vi "PH_Beckhoff_PPMA-Rods.handle Digital Inputs.vi"(0 "i ref in":refnum<vi>, 2 "States":T2(array[cluster]) {"Status" items=["no info", "off/false/out", "on/true/in", "Failure", "Alarm", "Status 1", "Status 2", "Status 3"]}, 3 "Digital Inputs":T3, 5 "error in":errorcluster) -> (14 "i ref out":refnum<vi>, 19 "error out":errorcluster)   [LabVIEW 2014, in "PH_Beckhoff_PPMA-Rods.lvlib"]
doc: "This VI sets the digital Input GUI elements which is whether the rods ar up or not."
uses:
  PH_Beckhoff_PPMA-Rods.lvlib
  PH_Beckhoff/PH_Beckhoff.Digital Inputs.ctl
  PH_Basics/PH_StatusHandler/PH_StatusHandler.Status.ctl
  PH_Basics/PH_StatusHandler/PH_StatusHandler.lvlib
  PH_Beckhoff/PH_Beckhoff.lvlib
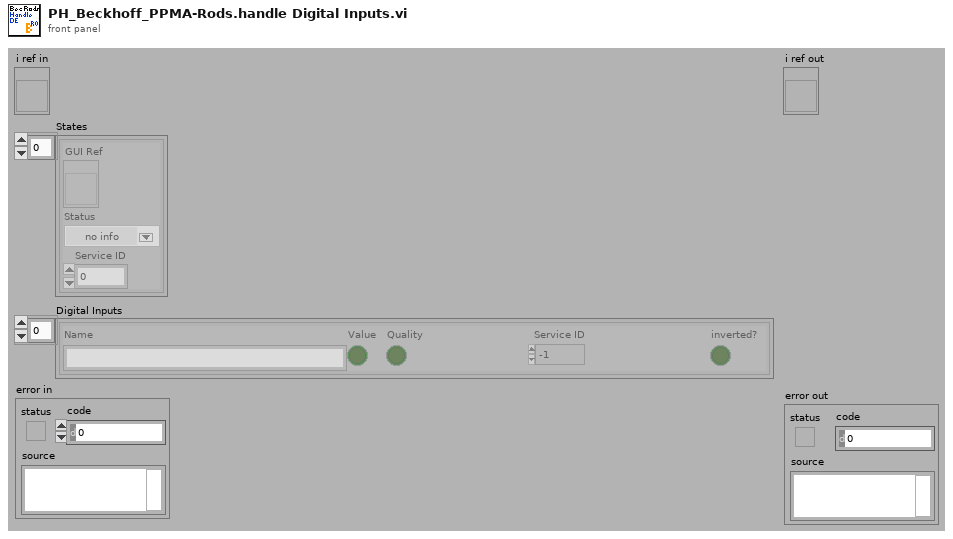
[diagram p1: front panel]
types:
  T1 = typedef "PH_StatusHandler.lvlib/PH_StatusHandler.Status.ctl" = i16
  T2 = cluster{"GUI Ref":refnum<vi>, "Status":T1, "Service ID":i32}[]
  T3 = typedef "PH_Beckhoff.lvlib/PH_Beckhoff.Digital Inputs.ctl" = cluster{"Name":string, "Value":bool, "Quality":bool, "Service ID":i32, "inverted?":bool}[]
  T4 = typedef "PH_Beckhoff_PPMA-Rods.lvlib/PH_Beckhoff_PPMA-Rods.i attribute.ctl" = cluster{"Input Up GUI Refs":refnum<vi>[], "Output GUI Refs":cluster{"Rod A up":refnum<vi>, "Rod B up":refnum<vi>, "Warnlamp orange":refnum<vi>, "Warnlamp green":refnum<vi>}, "States":cluster{"GUI Ref":refnum<vi>, "Status":T1, "Service ID":i32}[], "Input GUI Refs":cluster{"earth ok":refnum<vi>, "door locked K1":refnum<vi>, "door locked K2":refnum<vi>, "valve closed":refnum<vi>}}
  T5 = cluster{"GUI Ref":refnum<vi>, "Status":T1, "Service ID":i32}
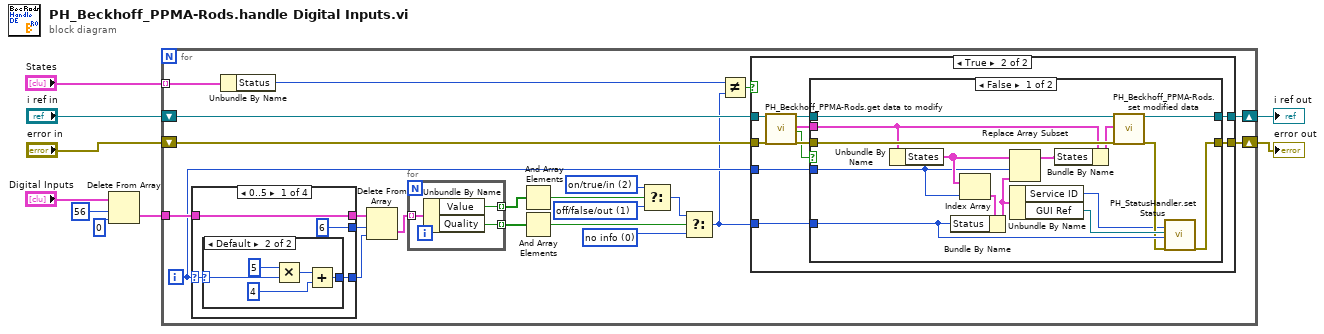
[diagram p0: block diagram]
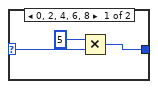
[diagram p4: hidden frame]
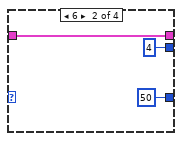
[diagram p5: hidden frame]
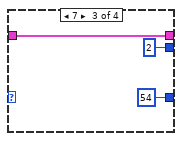
[diagram p6: hidden frame]
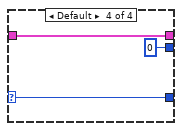
[diagram p7: hidden frame]
diagram:
  n1 = Delete From Array(array="Digital Inputs", length=56, index=0) -> (deleted portion=w1:T3)  [unwired: 1 out]
  n2 = for {
    shift-right: [w17] -> w7
    shift-left: "error in" -> [w31]
    tunnel: "States" -> [w30] mode=indexing
    tunnel: w1 -> [w29]
    shift-right: [w16] -> w3
    shift-left: "i ref in" -> [w15]
    i -> [w14]
    w19 = T1 1 items=["no info", "off/false/out", "on/true/in", "Failure", "Alarm", "Status 1", "Status 2", "Status 3"] ("f")
    w20 = T1 2 items=["no info", "off/false/out", "on/true/in", "Failure", "Alarm", "Status 1", "Status 2", "Status 3"] ("Status")
    w24 = T1 0 items=["no info", "off/false/out", "on/true/in", "Failure", "Alarm", "Status 1", "Status 2", "Status 3"] ("Status")
    n3 = case shown="0..5" w14 {
      selector: w14 -> [w64 _ _ w82]
      tunnel: w29 -> [w67 w78 w81 w84]
      tunnel: [w67 w78 w81 w84] -> w28
      tunnel: [6 ("length") 4 ("length") 2 ("length") 0 ("length")] -> w27
      tunnel: [w65 50 54 w82] -> w13
      frame 0..5 {
        n4 = case shown="Default" w64 {
          selector: w64 -> [w68 w74]
          tunnel: [w69 w73] -> w65
          frame 0, 2, 4, 6, 8 {
            n5 = Multiply(x=5 ("index"), y=w68) -> (x*y=w69:i32)
          }
          frame Default {
            n6 = Multiply(x=5 ("index"), y=w74) -> (x*y=w72:i32)
            n7 = Add(x=w72, y=4) -> (x+y=w73:i32)
          }
        }
      }
      frame 6 {
      }
      frame 7 {
      }
      frame Default {
      }
    }
    n8 = Unbundle By Name(w30) -> ("Status"=w18:T1)
    n9 = Delete From Array(array=w28, length=w27, index=w13) -> (deleted portion=w10:T3)  [unwired: 1 out]
    n10 = for {
      tunnel: w10 -> [w63] mode=indexing
      tunnel: [w62] -> w26 mode=indexing
      tunnel: [w61] -> w23 mode=indexing
      n11 = Unbundle By Name(w63) -> ("Value"=w61:bool, "Quality"=w62:bool)
    }
    n12 = And Array Elements(Boolean array=w23) -> (logical AND=w22:bool)
    n13 = And Array Elements(Boolean array=w26) -> (logical AND=w25:bool)
    n14 = Select(t=w20, s=w22, f=w19) -> (s? t:f=w21:T1)
    n15 = Select(t=w21, s=w25, f=w24) -> (s? t:f=w12:T1)
    n16 = Not Equal?(x=w18, y=w12) -> (x != y?=w11:bool)
    n17 = case shown="True" w11 {
      tunnel: w31 -> [w32 w43]
      tunnel: [w32 w41] -> w17
      tunnel: [w33 w39] -> w16
      tunnel: w15 -> [w33 w38]
      tunnel: w14 -> [_ w35]
      tunnel: w12 -> [_ w34]
      frame False {
      }
      frame True {
        n18 = call "PH_Beckhoff_PPMA-Rods.get data to modify.vi"("i ref in"=w38, "error in (no error)"=w43) -> ("i ref out"=w40:refnum<vi>, "i attribute"=w36:T4, "timed out"=w37:bool, "error out"=w42:errorcluster)  [unwired: 14 in]
        n19 = case shown="False" w37 {
          tunnel: w42 -> [w58 w59]
          tunnel: [w46 w59] -> w41
          tunnel: w40 -> [w57 w60]
          tunnel: [w56 w60] -> w39
          tunnel: w36 -> [w54 _]
          tunnel: w35 -> [w50 _]
          tunnel: w34 -> [w47 _]
          frame False {
            n20 = Unbundle By Name(w54) -> ("States"=w52:T2)
            n21 = Index Array(array=w52, index=w50) -> (element=w51:T5)
            n22 = Bundle By Name(cluster=w51, "Status"=w47) -> (w49:T5)
            n23 = Replace Array Subset(array=w52, new element=w49, index=w50) -> (w53:T2)
            n24 = Unbundle By Name(w49) -> ("Service ID"=w44:i32, "GUI Ref"=w48:refnum<vi>)
            n25 = Bundle By Name(cluster=w54, "States"=w53) -> (w55:T4)
            n26 = call "PH_Beckhoff_PPMA-Rods.set modified data.vi"("i ref in"=w57, "i attribute"=w55, "error in (no error)"=w58) -> ("i ref out"=w56:refnum<vi>, "error out"=w45:errorcluster)  [unwired: 15 in]
            n27 = call "PH_StatusHandler.set Status.vi"("Service ID Status"=w44, "Ring in"=w48, "Status"=w47, "error in (no error)"=w45) -> ("error out"=w46:errorcluster)  [unwired: 15 in]
          }
          frame True {
          }
        }
      }
    }
  }
  "error out" <- w7
  "i ref out" <- w3
